vi "Datalogger Main.vi"() -> ()   [LabVIEW 2020]
uses:
  sub VIs/Globals.vi
  src/MCP Server/MCP Server.lvlib
panel:
  out "Waveform Graph":dbl[][](graph)
  in  "Logging":bool
  in  "Stop":bool
  in  "active channels":bool[](array[boolean])=[FALSE, FALSE, FALSE, FALSE, FALSE]
  in  "Connected?":bool[](array[boolean])=[TRUE, FALSE, TRUE, TRUE, TRUE]
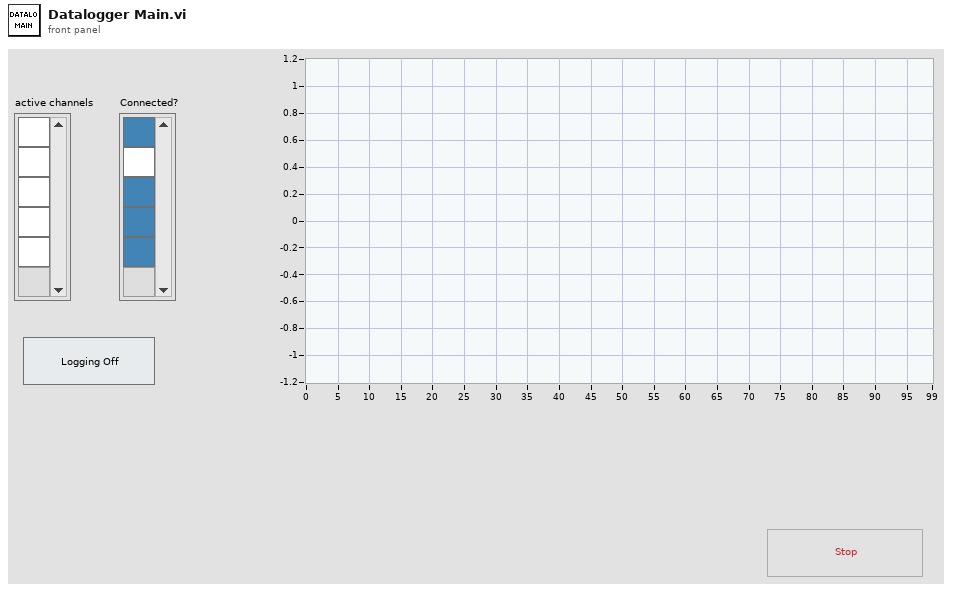
[diagram p1: front panel]
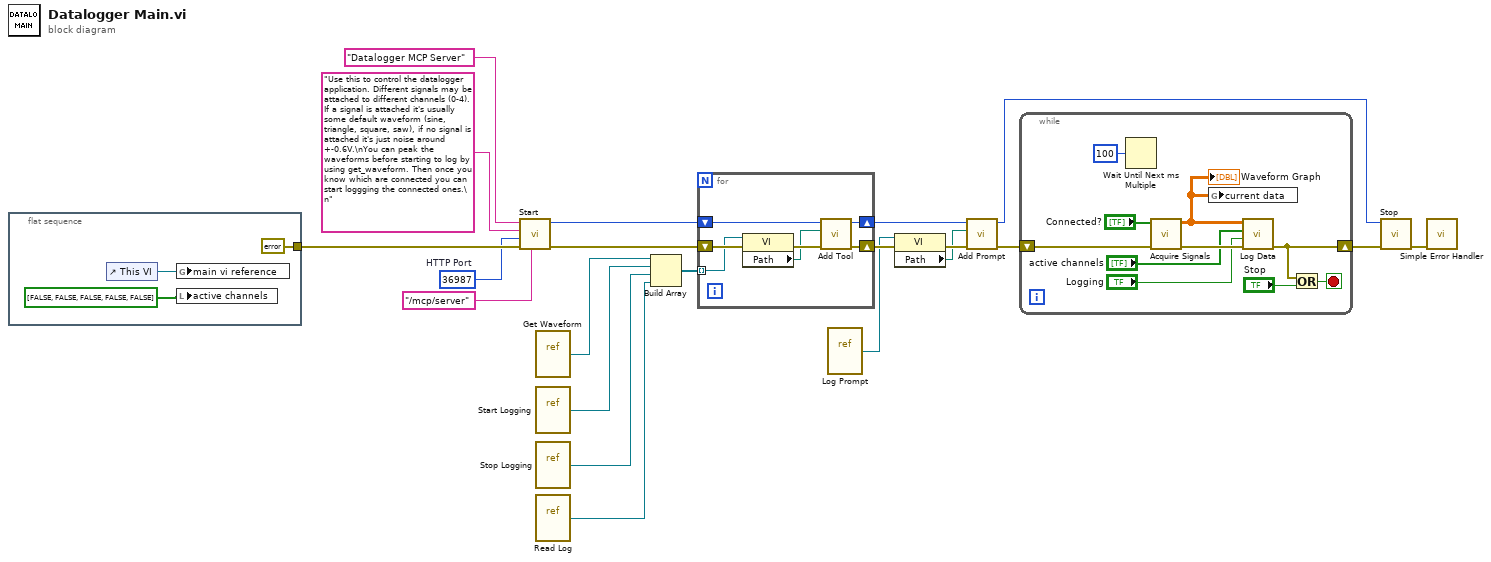
[diagram p0: block diagram]
diagram:
  w16 = u16 36987  # HTTP Port
  n1 = flat-sequence {
    tunnel: [errorcluster {"status"=FALSE, "code"=0, "source"=""} ("error out")] -> w20
    frame #0 {
      n2 = control-ref of="This VI"() -> (w24:refnum<vi>)
      n3 = global write "Globals.vi" "main vi reference"(w24) -> ()
      n4 = local write "active channels"(bool[] [FALSE, FALSE, FALSE, FALSE, FALSE] ("active channels")) -> ()
    }
  }
  n5 = call "Start.vi"("url (\"/mcp/server\")"="/mcp/server" ("url (\"/mcp/server\")"), "error in (no error)"=w20, "HTTP Port (36987)"=w16, "Description"="Use this to control the datalogger application. Different signals may be attached to different channels (0-4). If a signal is attached it's usually some default waveform (sine, triangle, square, saw), if no signal is attached it's just noise around +-0.6V.\nYou can peak the waveforms before starting to log by using get_waveform. Then once you know which are connected you can start loggging the connected ones.\n", "Name"="Datalogger MCP Server") -> ("error out"=w19:errorcluster, "server id out"=w13:i32)  [unwired: 4 in, 1 out]
  n6 = vi-ref "Get Waveform.vi"() -> (w11:refnum<vi>)
  n7 = vi-ref "Start Logging.vi"() -> (w9:refnum<vi>)
  n8 = vi-ref "Stop Logging.vi"() -> (w8:refnum<vi>)
  n9 = vi-ref "Read Log.vi"() -> (w7:refnum<vi>)
  n10 = Build Array(w11, w9, w8, w7) -> (w10:refnum<vi>[])
  n11 = for {
    shift-right: [w30] -> w14
    shift-left: w19 -> [w31]
    shift-right: [w28] -> w5
    shift-left: w13 -> [w29]
    tunnel: w10 -> [w26] mode=indexing
    n12 = property class="VI"(reference=w26, error in=w31) -> (error out=w27:errorcluster, "Path"=w25:path)  [unwired: 1 out]
    n13 = call "Add Tool.vi"("error in (no error)"=w27, "vi path"=w25, "server id"=w29) -> ("error out"=w30:errorcluster, "server id out"=w28:i32)  [unwired: 7 in]
  }
  n14 = vi-ref "Log Prompt.vi"() -> (w2:refnum<vi>)
  n15 = property class="VI"(reference=w2, error in=w14) -> (error out=w3:errorcluster, "Path"=w1:path)  [unwired: 1 out]
  n16 = call "Add Prompt.vi"("error in (no error)"=w3, "vi path"=w1, "server id"=w5) -> ("error out"=w6:errorcluster, "server id out"=w4:i32)  [unwired: 7 in]
  n17 = while {
    shift-right: [w33] -> w21
    shift-left: w6 -> [w38]
    stop <- w34 stop-if-true
    n18 = Wait Until Next ms Multiple(millisecond multiple=u32 100) -> ()  [unwired: 1 out]
    n19 = call "Acquire Signals.vi"("error in (no error)"=w38, "Connected?"="Connected?") -> ("error out"=w37:errorcluster, "Array"=w32:dbl[][])  [unwired: 8 in]
    "Waveform Graph" <- w32
    n20 = global write "Globals.vi" "current data"(w32) -> ()
    n21 = call "Log Data.vi"("error in (no error)"=w37, "Logging?"="Logging", "Channels to log"="active channels", "Array"=w32) -> ("error out"=w33:errorcluster)  [unwired: 7 in]
    n22 = Or(x=w33, y="Stop") -> (x .or. y?=w34:bool)
  }
  n23 = call "Stop.vi"("error in (no error)"=w21, "id"=w4) -> ("error out"=w12:errorcluster)  [unwired: 9 in]
  n24 = call <vilib>:"Simple Error Handler.vi"("error in (no error)"=w12) -> ()  [unwired: 4 in, 5 out]
